vi "Ctor.vi"(8 "error in (no error)":errorcluster, 11 "Dashboard Panel in":refnum<class "Dashboard Panel.lvclass">) -> (0 "error out":errorcluster, 3 "Dashboard Panel out":refnum<class "Dashboard Panel.lvclass">)   [LabVIEW 2020, in "SB App.lvlib" / "Dashboard Panel.lvclass"]
uses:
  Dashboard Panel.lvclass
  <vilib>/IlluminatedG/IG OOPanel/OOPanel/Panel/Panel.lvclass
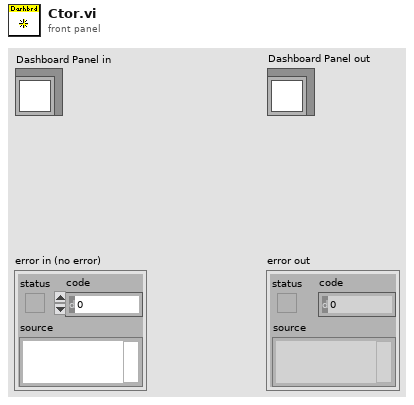
[diagram p1: front panel]
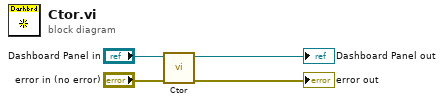
[diagram p0: block diagram]
diagram:
  n1 = call-parent "Ctor.vi"("error in (no error)"="error in (no error)", "Panel in"="Dashboard Panel in") -> ("error out"=→"error out":errorcluster, "Panel out"=→"Dashboard Panel out":refnum<class "Dashboard Panel.lvclass">)  [unwired: 8 in]
